vi "WS1050_36 DUT SData Ver1.0.vi"(0 "TMN DC\\CAP Data Log File Path":path=path "C:/temp", 1 "Lot#":string="WS1050", 2 "Total Delta C1(pF)":string[](array[string]), 3 "VSA_V1":string[][](array[string]), 4 "Wafer#":string="T7", 5 "File Name":string="Test Data", 6 "Total Delta C2(pF)":string[](array[string]), 7 "error in":errorcluster, 8 "TP/Comment":T1={"Test Program"="Multi Socket", "Comment"="HD_Cycling", "DVA"="", "EFUSE CAL"="", "CP HD/CYC"="", "VDD"="", "Duty Cycle"="", "V_Test(V)"="", "V_VPI(V)"="", "Freq(Hz)"="", "Board#"=""}, 9 "EFuse":string[](array[string])=["NC", "NC", "NC", "NC", "NC", "NC", "NC", "NC", "NC", "NC", "NC", "NC", "NC", "NC", "NC", "NC", "NC", "NC", "NC", "NC", "NC", "NC", "NC", "NC", "NC", "NC", "NC", "NC", "NC", "NC", "NC", "NC", "NC", "NC", "NC", "NC"], 10 "Data Output C3":string[][](table), 11 "Temperature":string="WS1033", 12 "VSA_V2":string[][](array[string]), 13 "VPI C3":string[][](array[string]), 14 "Data Output C1":string[][](table), 15 "VPI C2":string[][](array[string]), 16 "SN":string[](array[string])=["1", "2", "3", "4", "5", "6", "7", "8", "9", "10", "11", "12", "13", "14", "15", "16", "17", "18", "19", "20", "21", "22", "23", "24", "25", "26", "27", "28", "29", "30", "31", "32", "33", "34", "35", "36"], 17 "R/W Status":string[](array[string])=["PASS", "PASS", "PASS", "PASS", "PASS", "PASS", "PASS", "PASS", "PASS", "PASS", "PASS", "PASS", "PASS", "PASS", "PASS", "PASS", "PASS", "PASS", "PASS", "PASS", "PASS", "PASS", "PASS", "PASS", "PASS", "PASS", "PASS", "PASS", "PASS", "PASS", "PASS", "PASS", "PASS", "PASS", "PASS", "PASS"], 18 "Cap Header":string[](array[string]), 19 "Delta_RTZ_ Out":string[][](array[string]), 20 "HD/Cycles Completed":string="Test Data", 21 "Data Output C2":string[][](table), 23 "VSA_V3":string[][](array[string]), 24 "Current":string[](array[string]), 25 "VPI C1":string[][](array[string]), 26 "Total Delta C3(pF)":string[](array[string])) -> (27 "error out":errorcluster)   [LabVIEW 2012]
panel:
  in  "Bin":string[](array[string])=["NC", "NC", "NC", "NC", "NC", "NC", "NC", "NC", "NC", "NC", "NC", "NC", "NC", "NC", "NC", "NC", "NC", "NC", "NC", "NC", "NC", "NC", "NC", "NC", "NC", "NC", "NC", "NC", "NC", "NC", "NC", "NC", "NC", "NC", "NC", "NC"]
  # "*********** Do Not Remove ***********\nCompany:  WiSpry Inc\n20 Fairbanks Ste 198 Irvine CA 92618\n\nAuthor:  Andy V Tran\nCreated:  09/17/2014\nLabVIEW 2012 Suite\nTP:  Multi-Socket Save Data ver1.0\n*****************************************"
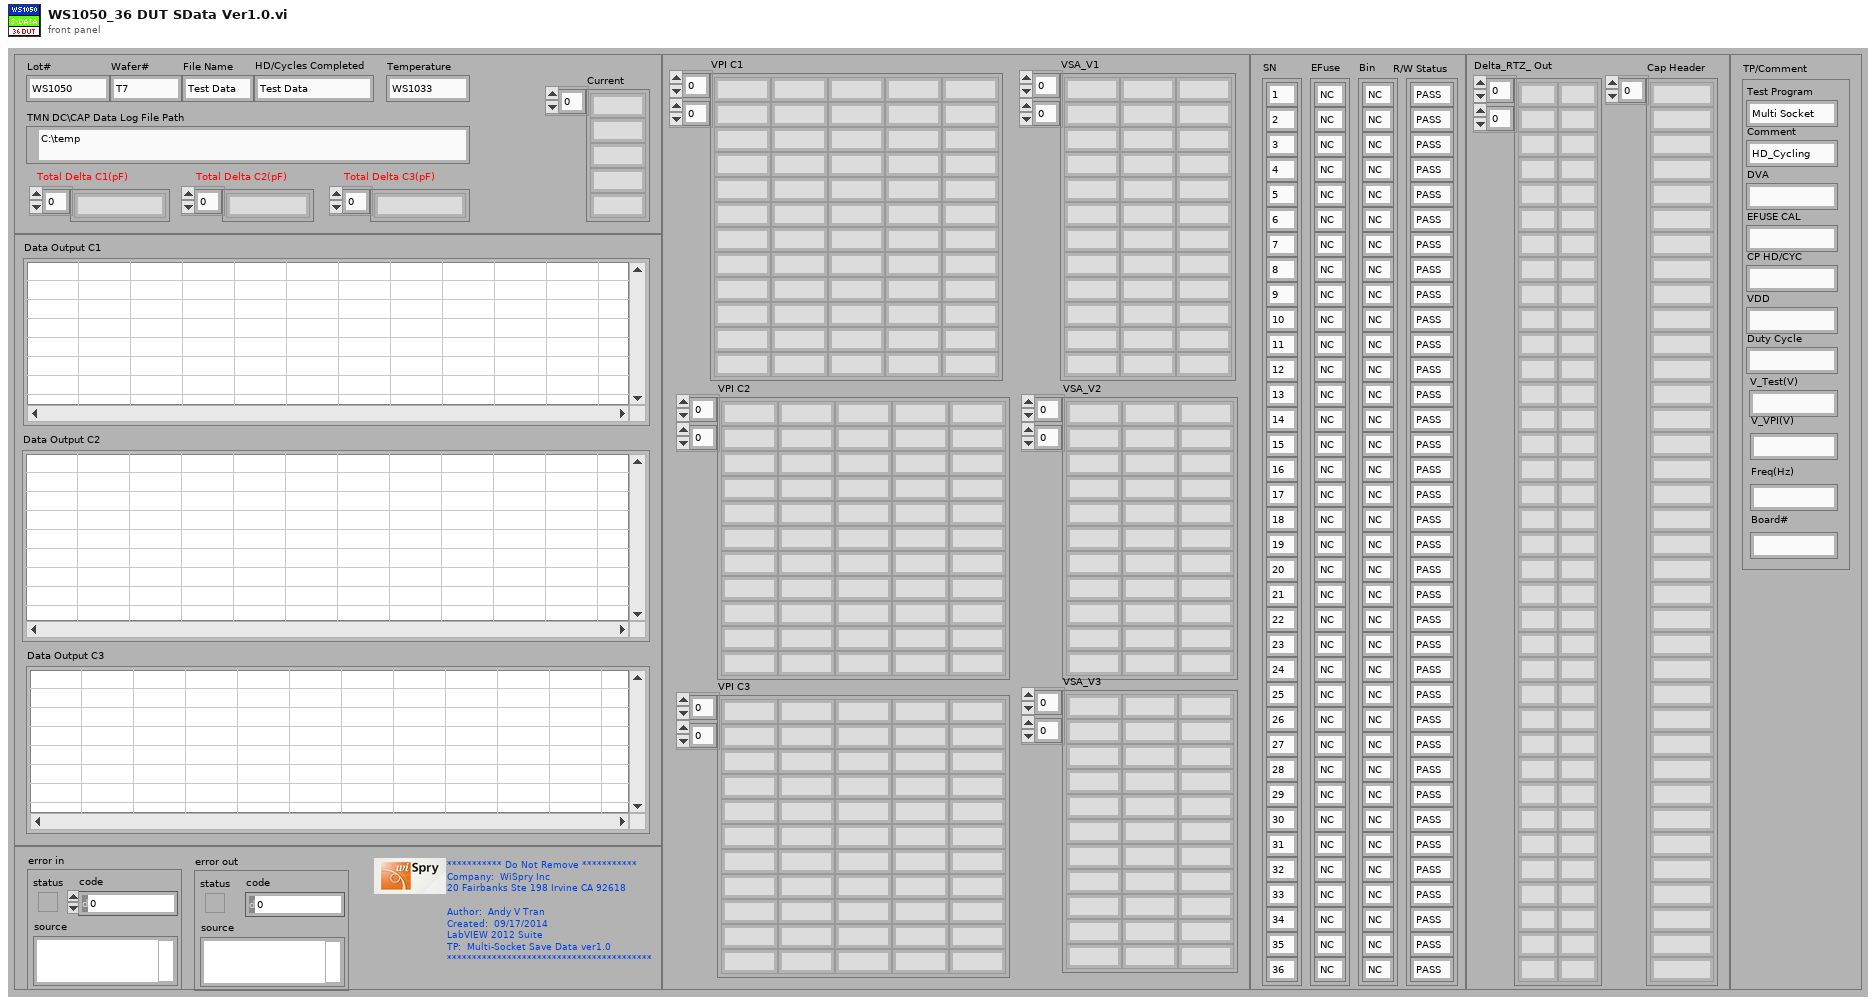
[diagram p1: front panel]
types:
  T1 = cluster{"Test Program":string, "Comment":string, "DVA":string, "EFUSE CAL":string, "CP HD/CYC":string, "VDD":string, "Duty Cycle":string, "V_Test(V)":string, "V_VPI(V)":string, "Freq(Hz)":string, "Board#":string}
  T2 = enum16{"open", "replace", "create", "open or create", "replace or create", "replace or create with confirmation"}
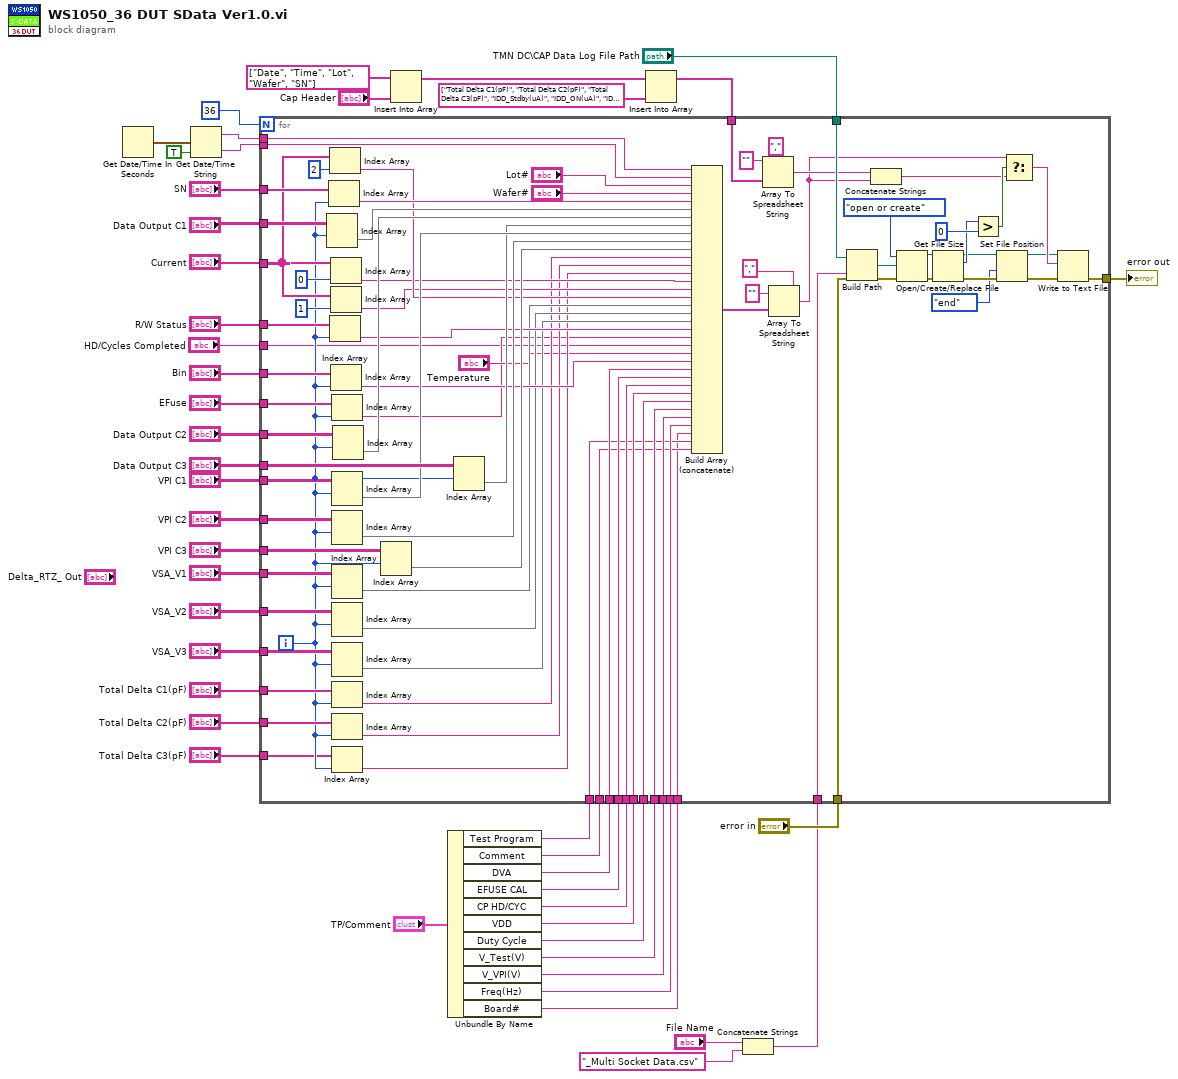
[diagram p0: block diagram]
diagram:
  n1 = Get Date/Time In Seconds() -> (seconds since 1Jan1904=w25:timestamp)
  n2 = Get Date/Time String(seconds (now)=w25, want seconds? (F)=TRUE) -> (date string=w33:string, time string=w34:string)  [unwired: 1 in]
  n3 = Insert Into Array(array=string[] ["Date", "Time", "Lot", "Wafer", "SN"], new element="Cap Header") -> (w11:string[])  [unwired: 1 in]
  n4 = Unbundle By Name("TP/Comment") -> ("Test Program"=w38:string, "Comment"=w37:string, "DVA"=w10:string, "EFUSE CAL"=w9:string, "CP HD/CYC"=w8:string, "VDD"=w7:string, "Duty Cycle"=w6:string, "V_Test(V)"=w5:string, "V_VPI(V)"=w4:string, "Freq(Hz)"=w2:string, "Board#"=w1:string)
  n5 = Insert Into Array(array=w11, new element=string[] ["Total Delta C1(pF)", "Total Delta C2(pF)", "Total Delta C3(pF)", "IDD_Stdby(uA)", "IDD_ON(uA)", "IDD_OFF(uA)", "VSA_V1_(V)", "VSA_V1_C1(pF)", "VSA_V1_C2(pF)", "VSA_V1_C3(pF)", "VSA_V2(V)", "VSA_V2_C1(pF)", "VSA_V2_C2(pF)", "VSA_V2_C3(pF)", "VSA_V3(V)", "VSA_V3_C1(pF)", "VSA_V3_C2(pF)", "VSA_V3_C3(pF)", "R/W Status(P/F)", "EFuse RB", "HD-CYC Completed", "Temperature", "Bin", "DVA ON/OFF", "CAL ON/OFF", "CP_HD/CYC", "VDD", "Duty Cycle(%)", "V_Test(V)", "V_VPI(V)", "Freq(Hz)", "Board", "Test Program", "Comment"]) -> (w15:string[])  [unwired: 1 in]
  n6 = Concatenate Strings("File Name", "_Multi Socket Data.csv" ("string")) -> (w41:string)
  n7 = for {
    N: 36 -> [_]
    tunnel: "TMN DC\\CAP Data Log File Path" -> [w129]
    tunnel: w15 -> [w128]
    tunnel: "error in" -> [w89]
    tunnel: w41 -> [w127]
    tunnel: [w105] -> w40
    tunnel: "SN" -> [w104]
    tunnel: "Current" -> [w96]
    tunnel: w38 -> [w48]
    tunnel: w37 -> [w49]
    tunnel: "Bin" -> [w103]
    tunnel: "R/W Status" -> [w102]
    tunnel: w34 -> [w79]
    tunnel: w33 -> [w78]
    tunnel: "Data Output C1" -> [w101]
    tunnel: "Data Output C2" -> [w100]
    tunnel: "VPI C1" -> [w95]
    tunnel: "VPI C2" -> [w94]
    tunnel: "EFuse" -> [w93]
    tunnel: "VSA_V1" -> [w92]
    tunnel: "VSA_V2" -> [w91]
    tunnel: "VSA_V3" -> [w90]
    tunnel: "VPI C3" -> [w88]
    tunnel: "Data Output C3" -> [w87]
    tunnel: "Total Delta C1(pF)" -> [w77]
    tunnel: "Total Delta C2(pF)" -> [w76]
    tunnel: "Total Delta C3(pF)" -> [w74]
    tunnel: w10 -> [w62]
    tunnel: w9 -> [w61]
    tunnel: w8 -> [w60]
    tunnel: w7 -> [w59]
    tunnel: w6 -> [w58]
    tunnel: w5 -> [w57]
    tunnel: w4 -> [w56]
    tunnel: "HD/Cycles Completed" -> [w51]
    tunnel: w2 -> [w50]
    tunnel: w1 -> [w47]
    i -> [w75]
    n8 = Index Array(array=w101, index (row)=w75) -> (element=w81:string[])  [unwired: 1 in]
    n9 = Index Array(array=w104, index=w75) -> (element=w80:string)
    n10 = Index Array(array=w96, index=2) -> (element=w68:string)
    n11 = Index Array(array=w102, index=w75) -> (element=w72:string)
    n12 = Index Array(array=w96, index=0) -> (element=w66:string)
    n13 = Index Array(array=w96, index=1) -> (element=w67:string)
    n14 = Index Array(array=w103, index=w75) -> (element=w73:string)
    n15 = Index Array(array=w93, index=w75) -> (element=w52:string)
    n16 = Index Array(array=w95, index (row)=w75) -> (element=w84:string[])  [unwired: 1 in]
    n17 = Index Array(array=w94, index (row)=w75) -> (element=w85:string[])  [unwired: 1 in]
    n18 = Index Array(array=w92, index (row)=w75) -> (element=w69:string[])  [unwired: 1 in]
    n19 = Index Array(array=w91, index (row)=w75) -> (element=w70:string[])  [unwired: 1 in]
    n20 = Index Array(array=w90, index (row)=w75) -> (element=w71:string[])  [unwired: 1 in]
    n21 = Index Array(array=w77, index=w75) -> (element=w65:string)
    n22 = Index Array(array=w76, index=w75) -> (element=w64:string)
    n23 = Index Array(array=w74, index=w75) -> (element=w63:string)
    n24 = Index Array(array=w100, index (row)=w75) -> (element=w82:string[])  [unwired: 1 in]
    n25 = Index Array(array=w88, index (row)=w75) -> (element=w86:string[])  [unwired: 1 in]
    n26 = Index Array(array=w87, index (row)=w75) -> (element=w83:string[])  [unwired: 1 in]
    n27 = Build Array (concatenate)(w78, w79, "Lot#", "Wafer#", w80, w81, w82, w83, w84, w85, w86, w65, w64, w63, w66, w67, w68, w69, w70, w71, w72, w52, w51, "Temperature", w73, w62, w61, w60, w59, w58, w57, w56, w50, w47, w48, w49) -> (w106:string[])
    n28 = Array To Spreadsheet String(delimiter (Tab)=",", array=w128, 3:"" ("format string")) -> (spreadsheet string=w109:string)
    n29 = Array To Spreadsheet String(delimiter (Tab)=",", array=w106, 3:"" ("format string")) -> (spreadsheet string=w107:string)
    n30 = Build Path(base path=w129, name or relative path=w127) -> (appended path=w121:path)
    n31 = Concatenate Strings(w109, w107) -> (w108:string)
    n32 = Open/Create/Replace File(file path (use dialog)=w121, error in=w89, operation (0:open)=T2."open or create") -> (refnum out=w119:refnum<file>, error out=w122:errorcluster)  [unwired: 4 out]
    n33 = Get File Size(file=w119, error in=w122) -> (refnum out=w114:refnum<file>, size (in bytes)=w118:i64, 0:w116:errorcluster)
    n34 = Greater?(x=w118, y=i64 0) -> (0:w123:bool)
    n35 = Set File Position(refnum=w114, from (0:start)=enum16{"start", "end", "current"}."end", error in=w116) -> (refnum out=w113:refnum<file>, error out=w115:errorcluster)  [unwired: 1 out]
    n36 = Select(t=w107, s=w123, f=w108) -> (s? t:f=w120:string)
    n37 = Write to Text File(file (use dialog)=w113, text=w120, error in=w115) -> (error out=w105:errorcluster)  [unwired: 3 out]
  }
  "error out" <- w40
